vi "Open.vi"(8 "error in (no error)":errorcluster, 11 "HAMAMATSU_DCAMAPI in":refnum<class "HAMAMATSU_DCAMAPI.lvclass">) -> (0 "error out":errorcluster, 3 "HAMAMATSU_DCAMAPI out":refnum<class "HAMAMATSU_DCAMAPI.lvclass">)   [LabVIEW 2020, in "HAMAMATSU_DCAMAPI.lvclass"]
uses:
  HAMAMATSU_DCAMAPI.lvclass
  HAMAMATSU_DCAMAPI.lvclass/HAMAMATSU_DCAMAPI.ctl
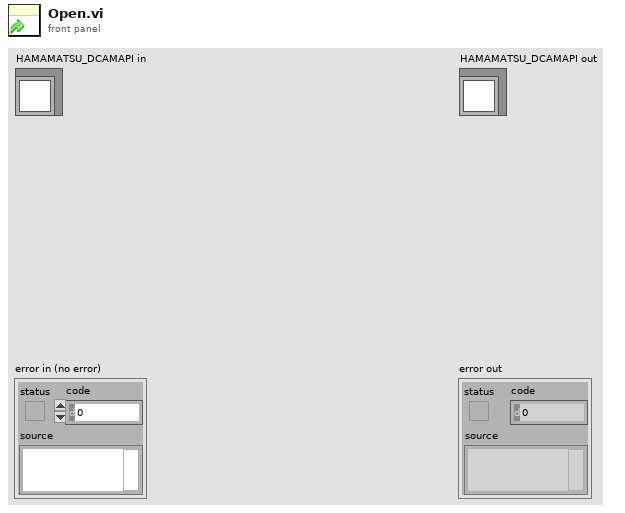
[diagram p1: front panel]
types:
  T1 = cluster{"Model":string, "Camera ID":string, "Firmware":string}
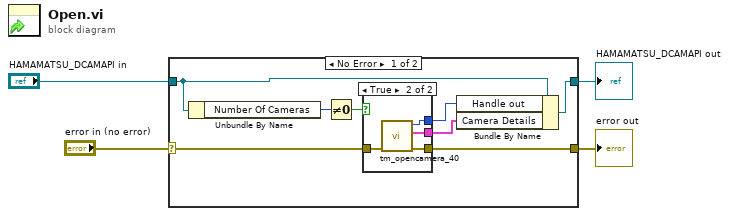
[diagram p0: block diagram]
diagram:
  n1 = case shown="No Error" "error in (no error)" {
    selector: "error in (no error)" -> [w6 w19]
    tunnel: "HAMAMATSU_DCAMAPI in" -> [w12 w18]
    tunnel: [w9 w18] -> w2
    tunnel: [w7 w19] -> w1
    frame No Error {
      n2 = Unbundle By Name(w12) -> ("Number Of Cameras"=w11:u32)
      n3 = Not Equal To 0?(x=w11) -> (x != 0?=w10:bool)
      n4 = case shown="True" w10 {
        tunnel: [_ w17] -> w8
        tunnel: [w13 w15] -> w7
        tunnel: w6 -> [w13 w16]
        tunnel: [_ w14] -> w5
        frame False {
        }
        frame True {
          n5 = call <userlib>:"tm_opencamera_40.vi"("error in (no error)"=w16) -> ("error out"=w15:errorcluster, "Camera Details"=w14:T1, "Handle out"=w17:u32)  [unwired: 8 in]
        }
      }
      n6 = Bundle By Name(cluster=w12, "Handle out"=w8, "Camera Details"=w5) -> (w9:refnum<class "HAMAMATSU_DCAMAPI.lvclass">)
    }
    frame Error {
    }
  }
  "error out" <- w1
  "HAMAMATSU_DCAMAPI out" <- w2
